vi "Write Data in tdms.vi"(7 "Command":T1, 8 "error in (no error)":errorcluster, 11 "Channel name":string[](array[string])) -> (0 "error out":errorcluster)   [LabVIEW 2021, in "ARINC.lvlib"]
uses:
  ARINC.lvlib
  Write Command.ctl
  User Interface/Create Path Command.ctl
  User Interface/User Interface.lvlib
panel:
  in  "Data":string[](array[string])
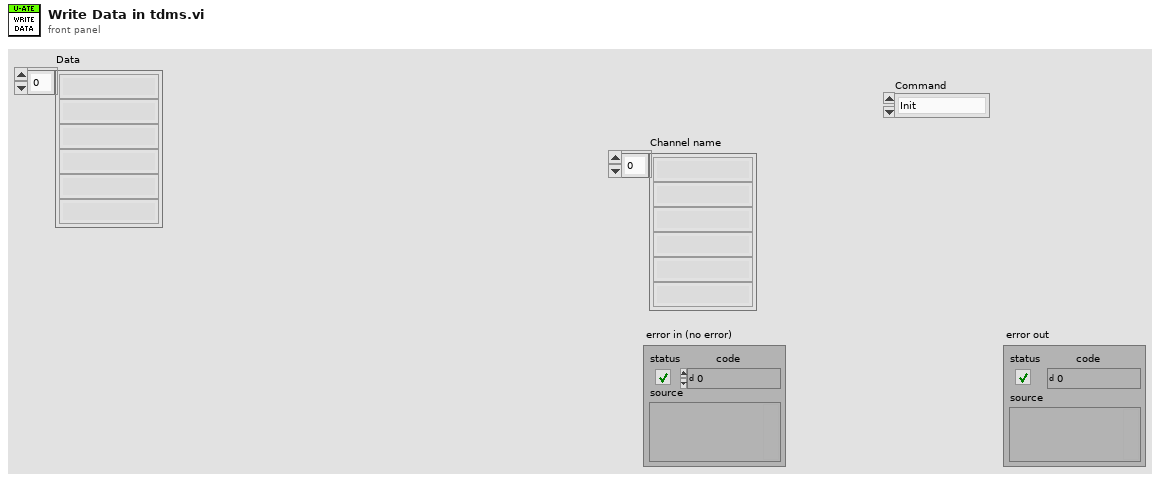
[diagram p1: front panel]
types:
  T1 = typedef "ARINC.lvlib/Write Command.ctl" = enum16{"Init", "Read", "Write", "Close"}
  T2 = typedef "User Interface.lvlib/Create Path Command.ctl" = enum16{"Authentication", "Hardware", "Configuration", "Calibration", "Instrument", "Test Description", "Serial Data", "ARINC Data", "CAN Data", "Data", "Report", "Action log", "Error Log"}
  T3 = enum16{"open", "open or create", "create or replace", "create", "open (read-only)"}
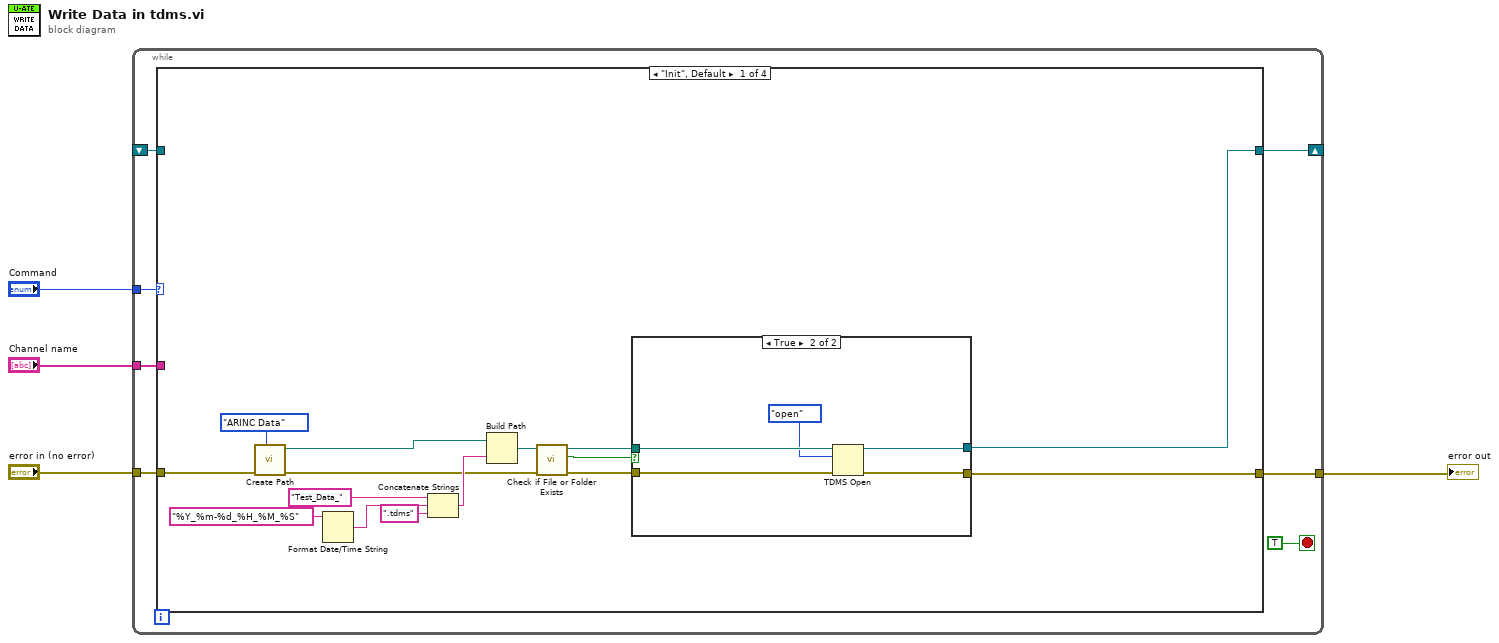
[diagram p0: block diagram]
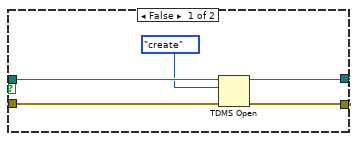
[diagram p2: hidden frame]
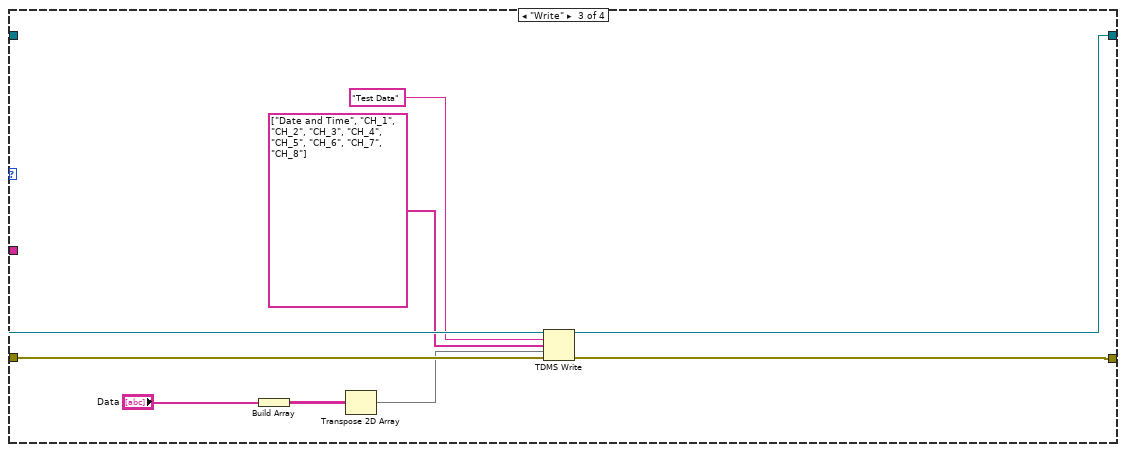
[diagram p4: hidden frame]
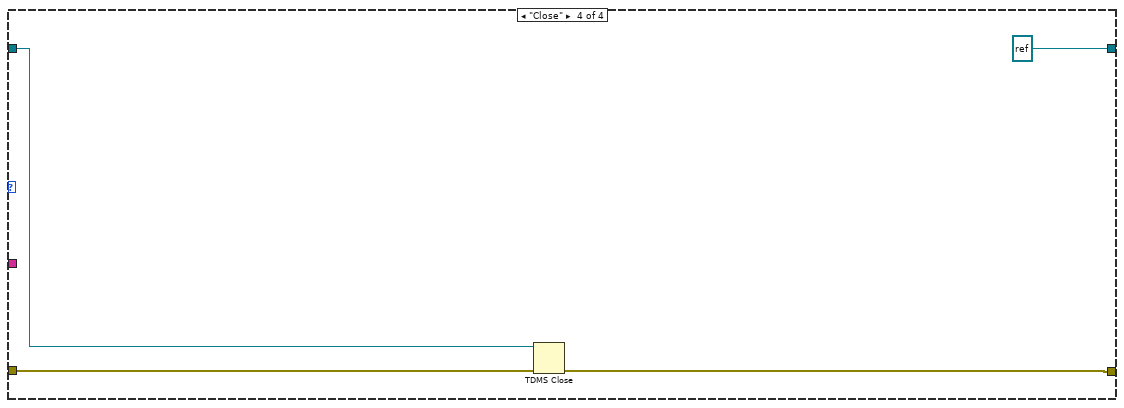
[diagram p5: hidden frame]
diagram:
  n1 = while {
    tunnel: "error in (no error)" -> [w10]
    tunnel: [w9] -> w3
    shift-right: [w8] -> _
    shift-left: _ -> [w7]
    tunnel: "Channel name" -> [w6]
    tunnel: "Command" -> [w5]
    stop <- TRUE stop-if-true
    n2 = case shown="\"Init\", Default" w5 {
      tunnel: w10 -> [w26 w37 w47 w51]
      tunnel: [w14 w37 w44 w50] -> w9
      tunnel: [w13 w38 w45 refnum<k34> refnum ("tdms file out")] -> w8
      tunnel: w7 -> [_ w38 w46 w49]
      tunnel: w6 -> [_ _ _ _]
      frame "Init", Default {
        n3 = call "Create Path.vi"("Path Command"=Create_Path_Command."ARINC Data", "error in (no error)"=w26) -> ("error out"=w15:errorcluster, "created path"=w21:path)  [unwired: 8 in]
        n4 = Format Date/Time String(time format string (%c)="%Y_%m-%d_%H_%M_%S") -> (date/time string=w19:string)  [unwired: 2 in]
        n5 = Concatenate Strings("Test_Data_" ("string"), w19, ".tdms" ("string")) -> (w17:string)
        n6 = Build Path(base path=w21, name or relative path=w17) -> (appended path=w16:path)
        n7 = call <vilib>:"Check if File or Folder Exists.vi"("error in (no error)"=w15, "path"=w16) -> ("error out"=w25:errorcluster, "file or folder exists?"=w24:bool, "dup path"=w23:path)  [unwired: 7 in]
        n8 = case shown="True" w24 {
          tunnel: w25 -> [w30 w36]
          tunnel: w23 -> [w31 w35]
          tunnel: [w28 w33] -> w14
          tunnel: [w27 w34] -> w13
          frame False {
            n9 = TDMS Open(8:w30, 10:T3."create" ("operation (0:open)"), 11:w31) -> (0:w28:errorcluster, 3:w27:refnum<k34>)  [unwired: 4 in]
          }
          frame True {
            n10 = TDMS Open(8:w36, 10:T3."open" ("operation (0:open)"), 11:w35) -> (0:w33:errorcluster, 3:w34:refnum<k34>)  [unwired: 4 in]
          }
        }
      }
      frame "Read" {
      }
      frame "Write" {
        n11 = Build Array("Data") -> (w40:string[][])
        n12 = Transpose 2D Array(2D array=w40) -> (transposed array=w39:string[][])
        n13 = TDMS Write(0:w46, 5:"Test Data", 7:string[] ["Date and Time", "CH_1", "CH_2", "CH_3", "CH_4", "CH_5", "CH_6", "CH_7", "CH_8"], 9:w39, 11:w47) -> (4:w45:refnum<k34>, 15:w44:errorcluster)  [unwired: 1 in, 2 out]
      }
      frame "Close" {
        n14 = TDMS Close(8:w51, 11:w49) -> (0:w50:errorcluster)  [unwired: 1 out]
      }
    }
  }
  "error out" <- w3
